vi "XML getApiResponses.vi"(10 "Responses In":T1[](array[typedef]), 11 "Responses XML":string) -> (2 "Responses Out":T1[](array[typedef]))   [LabVIEW 2011]
uses:
  Controls/PIM.API.Response.Unique.ctl
  Controls/PIM.API.Response.Samples.ctl
  iQA Sweep Behavior.ctl
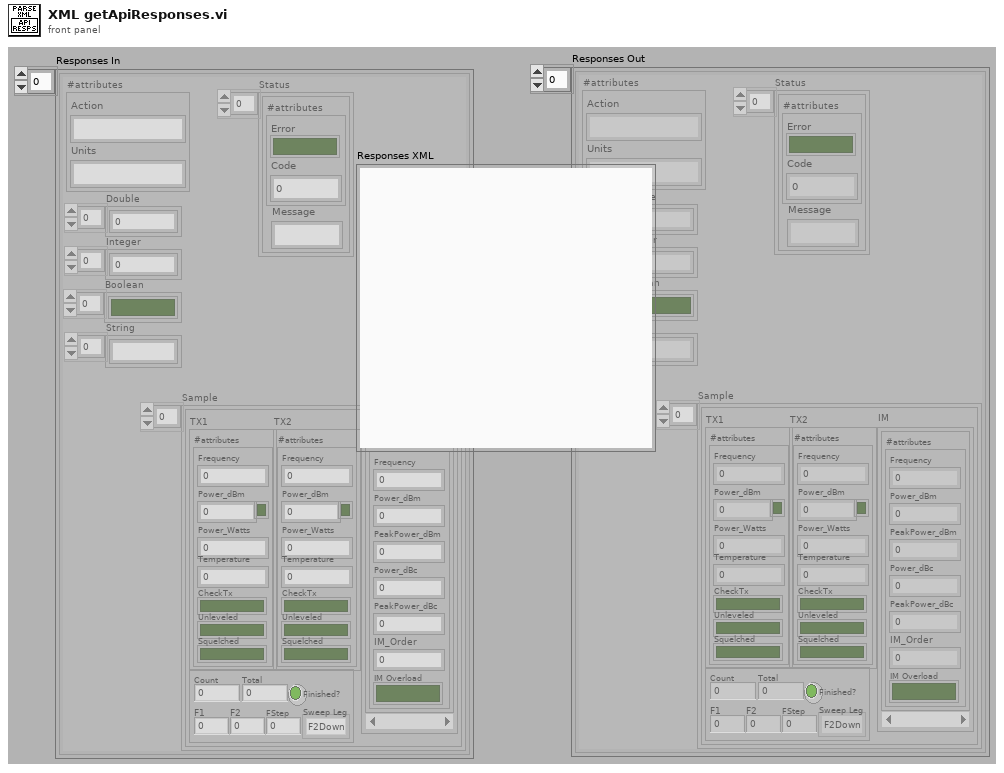
[diagram p1: front panel]
types:
  T1 = typedef "PIM.API.Response.Unique.ctl" = cluster{"#attributes":cluster{"Action":string, "Units":string}, "Double":dbl[], "Integer":i32[], "Boolean":bool[], "String":string[], "Sample":T2[], "Status":cluster{"#attributes":cluster{"Error":bool, "Code":i32}, "Message":string}[]}
  T2 = typedef "PIM.API.Response.Samples.ctl" = cluster{"TX1":cluster{"#attributes":cluster{"Frequency":dbl, "Power_dBm":dbl, "Power_Watts":dbl, "CheckTx":bool, "Unleveled":bool, "Squelched":bool, "Temperature":dbl, "ToneOn":bool}}, "TX2":cluster{"#attributes":cluster{"Frequency":dbl, "Power_dBm":dbl, "Power_Watts":dbl, "CheckTx":bool, "Unleveled":bool, "Squelched":bool, "Temperature":dbl, "ToneOn":bool}}, "IM":cluster{"#attributes":cluster{"Frequency":dbl, "Power_dBm":dbl, "PeakPower_dBm":dbl, "Power_dBc":dbl, "PeakPower_dBc":dbl, "IM_Order":u8, "IM Overload":bool}}[], "#attributes":cluster{"Count":u32, "Total":u32, "Finished?":bool, "Sweep Leg":T3, "F1":dbl, "F2":dbl, "FStep":dbl}}
  T3 = typedef "iQA Sweep Behavior.ctl" = enum16{"F2Down", "F1Up", "RxMultiIM"}
  T4 = cluster{"#attributes":cluster{"Error":bool, "Code":i32}, "Message":string}
  T5 = cluster{"#attributes":cluster{"Error":bool, "Code":i32}, "Message":string}[]
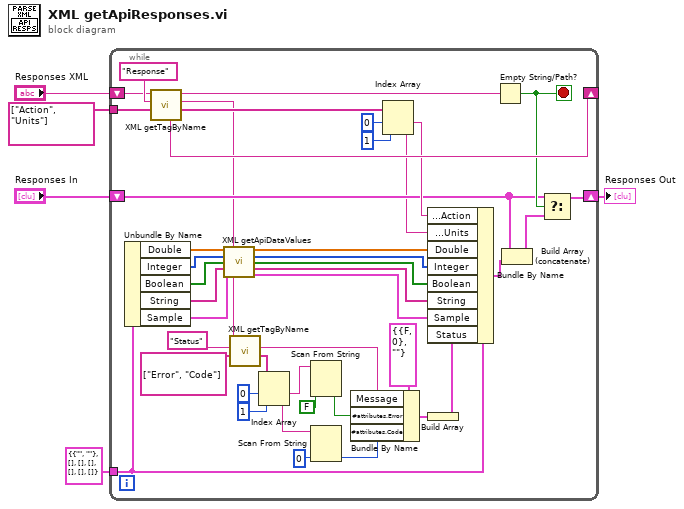
[diagram p0: block diagram]
diagram:
  n1 = while {
    shift-right: [w45] -> _
    shift-left: "Responses XML" -> [w46]
    shift-right: [w41] -> w5
    shift-left: "Responses In" -> [w38]
    tunnel: T1 {"#attributes"={"Action"="", "Units"=""}, "Double"=[], "Integer"=[], "Boolean"=[], "String"=[], "Sample"=[], "Status"=[]} -> [w35]
    tunnel: string[] ["Action", "Units"] -> [w39]
    stop <- w40 stop-if-true
    n2 = Unbundle By Name(w35) -> ("Double"=w34:dbl[], "Integer"=w33:i32[], "Boolean"=w32:bool[], "String"=w31:string[], "Sample"=w6:T2[])
    n3 = call "XML getTagByName.vi"("Get Attributes"=w39, "Tag Name"="Response", "XML String"=w46) -> ("Attribute Values"=w42:string[], "Tag Contents"=w22:string, "Matching Tag"=w44:string, "After Tag"=w45:string)  [unwired: 4 in, 1 out]
    n4 = call "XML getApiDataValues.vi"("Double in"=w34, "XML Data"=w22, "Integer in"=w33, "Boolean in"=w32, "String in"=w31, "Sample in"=w6) -> ("Double out"=w30:dbl[], "Integer out"=w29:i32[], "Boolean out"=w28:bool[], "String out"=w27:string[], "Sample out"=w7:T2[])  [unwired: 5 in]
    n5 = call "XML getTagByName.vi"("Get Attributes"=string[] ["Error", "Code"], "Tag Name"="Status", "XML String"=w22) -> ("Attribute Values"=w13:string[], "Tag Contents"=w18:string)  [unwired: 4 in, 3 out]
    n6 = Index Array(array=w13, index #1=0 ("index"), index #2=1 ("index")) -> (element #1=w12:string, element #2=w9:string)
    n7 = Scan From String(input string=w12, default 1=FALSE) -> (output 1=w11:bool)  [unwired: 3 in, 3 out]
    n8 = Scan From String(input string=w9, default 1=0 ("index")) -> (output 1=w8:i32)  [unwired: 3 in, 3 out]
    n9 = Bundle By Name(cluster=T4 {"#attributes"={"Error"=FALSE, "Code"=0}, "Message"=""}, "Message"=w18, "#attributes.Error"=w11, "#attributes.Code"=w8) -> (w17:T4)
    n10 = Index Array(array=w42, index #1=0 ("index"), index #2=1 ("index")) -> (element #1=w43:string, element #2=w24:string)
    n11 = Build Array(w17) -> (w16:T5)
    n12 = Bundle By Name(cluster=w35, "#attributes.Action"=w43, "#attributes.Units"=w24, "Double"=w30, "Integer"=w29, "Boolean"=w28, "String"=w27, "Sample"=w7, "Status"=w16) -> (w37:T1)
    n13 = Empty String/Path?(string/path=w44) -> (empty?=w40:bool)
    n14 = Build Array (concatenate)(w38, w37) -> (w36:T1[])
    n15 = Select(t=w38, s=w40, f=w36) -> (s? t:f=w41:T1[])
  }
  "Responses Out" <- w5
